vi "close configuration.vi"(8 "error in (no error)":errorcluster, 11 "named node map":refnum<k20>) -> (0 "error out":errorcluster)   [LabVIEW 2012, in "CreateOPCUAServerAuto.lvlib"]
uses:
  <vilib>/xml/Close Reference(NNMap).vi
  CreateOPCUAServerAuto.lvlib
  <vilib>/xml/NI_XML.lvlib
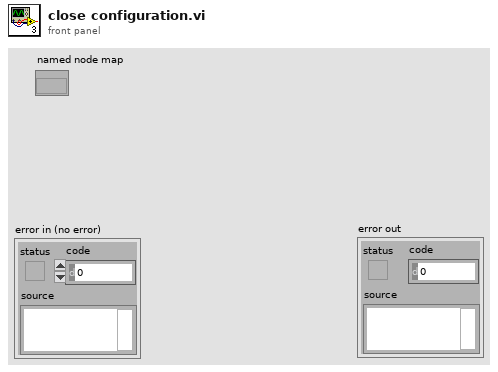
[diagram p1: front panel]
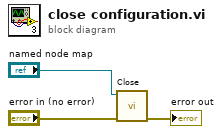
[diagram p0: block diagram]
diagram:
  n1 = call-poly <vilib>:"Close.vi"("error in (no error)"="error in (no error)", "named node map"="named node map") -> ("error out"=→"error out":errorcluster)  [unwired: 7 out]
